vi "Subvi Select Directory.vi"(0 "Prompt":string) -> (1 "FullFileName":string, 2 "Dir Name":string, 3 "Cancelled":bool)   [LabVIEW 2012]
doc: "This VI Sets the Image File Name and allows the user to create/select the directory of choice. Returns Full Path to the File Name and Directory chosen."
uses:
  ProSCI Global.vi
panel:
  in  "CancelButton":bool
  in  "OKButton":bool
  out "CurrentDir":string="C:\\"
  in  "SelDirectory":bool
  in  "FileName":string
  # "Present Image File Directory"
  # "Image File Name (no extension)"
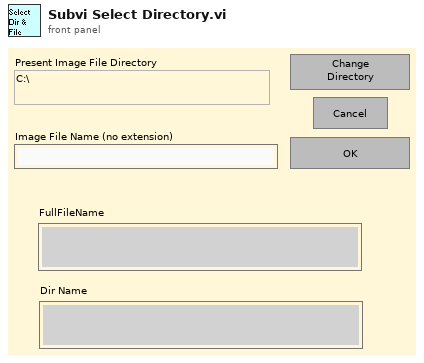
[diagram p1: front panel]
types:
  T1 = enum32{"existing file", "new file", "new or existing file", "existing dir", "new dir", "new or existing dir", "existing file (use LLBs)", "new file (use LLBs)", "new or existing file (use LLBs)", "new or existing file or directory (use LLBs)"}
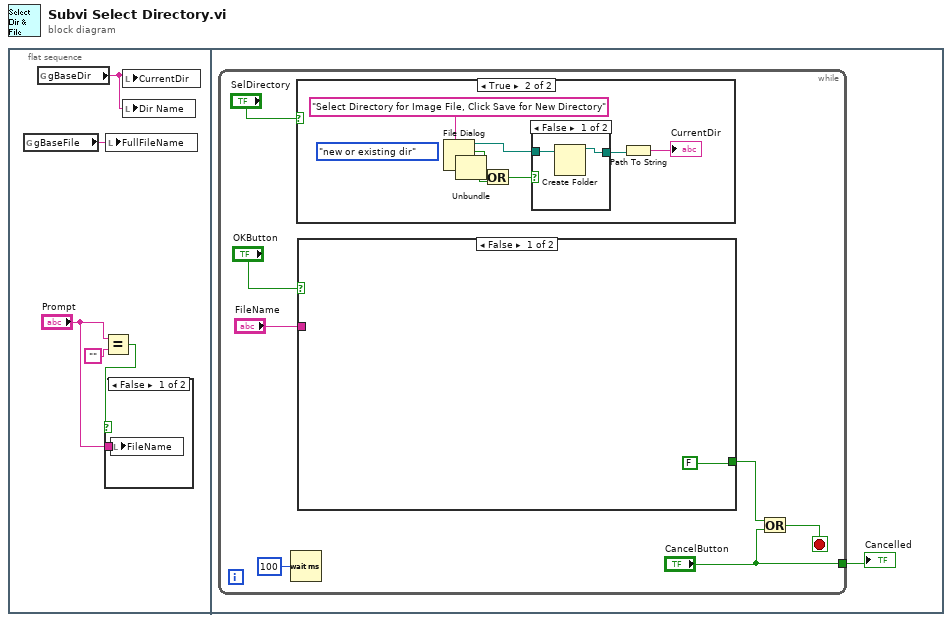
[diagram p0: block diagram]
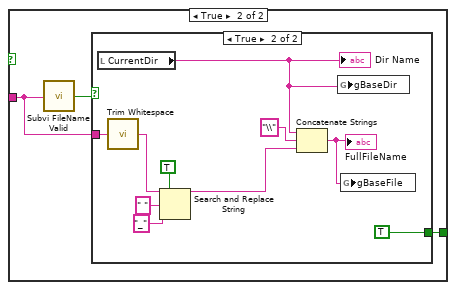
[diagram p3: hidden frame]
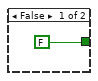
[diagram p4: hidden frame]
diagram:
  n1 = flat-sequence {
    frame #0 {
      n2 = global read "ProSCI Global.vi" "gBaseFile"() -> (w1:string)
      n3 = global read "ProSCI Global.vi" "gBaseDir"() -> (w2:string)
      n4 = Equal?(x="Prompt", y="") -> (x = y?=w4:bool)
      n5 = case shown="False" w4 {
        tunnel: "Prompt" -> [w6 _]
        frame False {
          n6 = local write "FileName"(w6) -> ()
        }
        frame True {
        }
      }
      n7 = local write "FullFileName"(w1) -> ()
      n8 = local write "CurrentDir"(w2) -> ()
      n9 = local write "Dir Name"(w2) -> ()
    }
    frame #1 {
      n10 = while {
        tunnel: ["CancelButton"] -> w7
        stop <- w9 stop-if-true
        n11 = Wait (ms)(milliseconds to wait=u32 100) -> ()  [unwired: 1 out]
        n12 = case shown="True" "SelDirectory" {
          frame False {
          }
          frame True {
            (unwired) T1."new or existing dir" ("select mode (2)")
            n13 = File Dialog(7:"Select Directory for Image File, Click Save for New Directory" ("prompt")) -> (0:w30:errorcluster, 1:w35:bool, 2:w36:bool, 3:w33:path)  [unwired: 1 in, 5 out]
            n14 = Unbundle(w30) -> ()  [unwired: 3 out]
            n15 = Or(x=w36, y=w35) -> (x .or. y?=w34:bool)
            n16 = case shown="False" w34 {
              tunnel: w33 -> [w39 w40]
              tunnel: [w38 w40] -> w32
              frame False {
                n17 = Create Folder(path (use dialog)=w39) -> (created path=w38:path)  [unwired: 1 in, 3 out]
              }
              frame True {
              }
            }
            n18 = Path To String(path=w32) -> (string=→"CurrentDir":string)
          }
        }
        n19 = case shown="False" "OKButton" {
          tunnel: "FileName" -> [_ w17]
          tunnel: [FALSE w16] -> w10
          frame False {
          }
          frame True {
            n20 = call "Subvi FileName Valid.vi"("InFileName"=w17) -> ("Success"=w18:bool)
            n21 = case shown="True" w18 {
              tunnel: w17 -> [_ w26]
              tunnel: [FALSE TRUE] -> w16
              frame False {
              }
              frame True {
                n22 = local read "CurrentDir"() -> (w27:string)
                "Dir Name" <- w27
                n23 = call <vilib>:"Trim Whitespace.vi"("string"=w26) -> ("trimmed string"=w22:string)  [unwired: 1 in]
                n24 = Search and Replace String(replace all?=TRUE ("replace all? (F)"), input string=w22, search string=" ", replace string="_" ("replace string (\"\")")) -> (result string=w21:string)  [unwired: 1 in, 6 out]
                n25 = Concatenate Strings(w27, "\\" ("string"), w21) -> (w29:string)
                "FullFileName" <- w29
                n26 = global write "ProSCI Global.vi" "gBaseDir"(w27) -> ()
                n27 = global write "ProSCI Global.vi" "gBaseFile"(w29) -> ()
              }
            }
          }
        }
        n28 = Or(x=w10, y="CancelButton") -> (x .or. y?=w9:bool)
      }
      "Cancelled" <- w7
    }
  }
